vi "FT10_Unitherm Clear Load.vi"(8 "error in (no error)":errorcluster, 11 "VISA Refnum in":refnum<visa-resource-name>) -> (0 "error out":errorcluster, 3 "VISA Refnum out":refnum<visa-resource-name>)   [LabVIEW 2024]
doc: "Changes resistance on Unitherm to 0 Ohms"
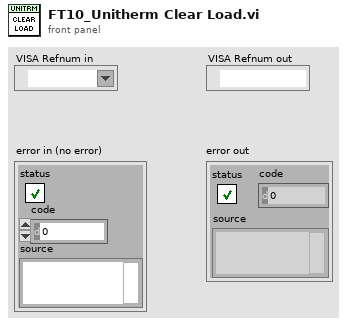
[diagram p1: front panel]
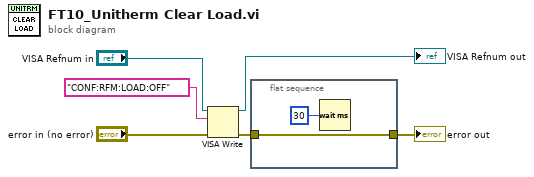
[diagram p0: block diagram]
diagram:
  n1 = VISA Write(VISA resource name="VISA Refnum in", write buffer="CONF:RFM:LOAD:OFF" ("string"), error in (no error)="error in (no error)") -> (VISA resource name out=→"VISA Refnum out":refnum<visa-resource-name>, error out=w5:errorcluster)  [unwired: 1 out]
  n2 = flat-sequence {
    tunnel: w5 -> [w7]
    tunnel: [w7] -> w6
    frame #0 {
      n3 = Wait (ms)(milliseconds to wait=u32 30) -> ()  [unwired: 1 out]
    }
  }
  "error out" <- w6
